vi "convert data type string to enum.vi"(8 "error in":errorcluster, 11 "Data Type String":string) -> (0 "error out":errorcluster, 3 "Data Type Enum":T1)   [LabVIEW 2013, in "control module configuration.lvclass"]
uses:
  control module configuration.lvclass
  <vilib>/NI/Tag Bus/tag/Data Type.ctl
  <vilib>/NI/Tag Bus/tag/tag descriptor.lvclass
  <vilib>/NI/Configuration Framework/NISE_CEF_TreeControl.lvlib
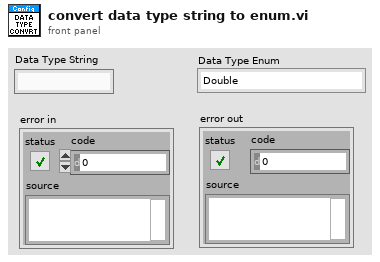
[diagram p1: front panel]
types:
  T1 = typedef "tag bus.lvlib/tag descriptor.lvclass/Data Type.ctl" = enum16{"Double", "Single", "I64", "I32", "I16", "I8", "U64", "U32", "U16", "U8", "Boolean", "String", "Array of Double", "Array of Single", "Array of I64", "Array of I32", "Array of I16", "Array of I8", "Array of U64", "Array of U32", "Array of U16", "Array of U8", "Array of Boolean", "Array of String"}
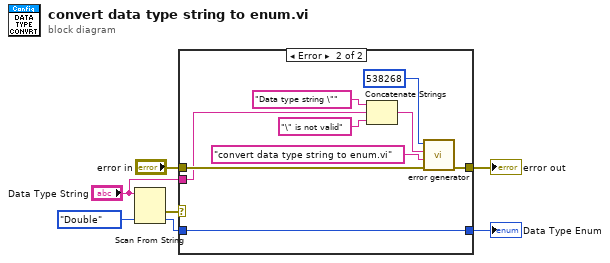
[diagram p0: block diagram]
diagram:
  n1 = Scan From String(input string="Data Type String", default 1=Data_Type."Double" ("Data Type Enum 2")) -> (error out=w4:errorcluster, output 1=w1:T1)  [unwired: 3 in, 2 out]
  n2 = case shown="Error" w4 {
    tunnel: "Data Type String" -> [_ w12]
    tunnel: [w8 w16] -> w6
    tunnel: w1 -> [w9 w18]
    tunnel: [w9 w18] -> w5
    tunnel: "error in" -> [w8 w17]
    frame No Error {
    }
    frame Error {
      n3 = Concatenate Strings("Data type string \"" ("source"), w12, "\" is not valid" ("string")) -> (w11:string)
      n4 = call <vilib>:"error generator.vi"("error in"=w17, "source"="convert data type string to enum.vi", "append error message"=w11, "error code (0)"=538268) -> ("error out"=w16:errorcluster)  [unwired: 5 in]
    }
  }
  "error out" <- w6
  "Data Type Enum" <- w5
